vi "nRF52 DK Generate Packets.vi"() -> ()   [LabVIEW 2026, in "Nordic nRF52 DK DTM Test.lvlib"]
uses:
  Nordic nRF52 DK DTM Test.lvlib
  PacketType.ctl
  TxRx.ctl
panel:
  out "error out":errorcluster
  in  "stop":bool
  in  "Tx Packet Type":T1
  in  "BLE Channel Number (0-39)":u8
  in  "Com Port Resource":refnum<visa-resource-name>="COM3"
  in  "Baud Rate":u32=19200
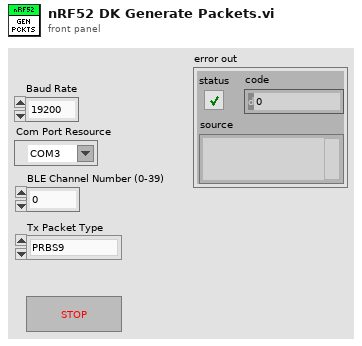
[diagram p1: front panel]
types:
  T1 = typedef "Nordic nRF52 DK DTM Test.lvlib/PacketType.ctl" = enum16{"PRBS9", "DF1", "DF2"}
  T2 = typedef "Nordic nRF52 DK DTM Test.lvlib/TxRx.ctl" = enum16{"Tx", "Rx"}
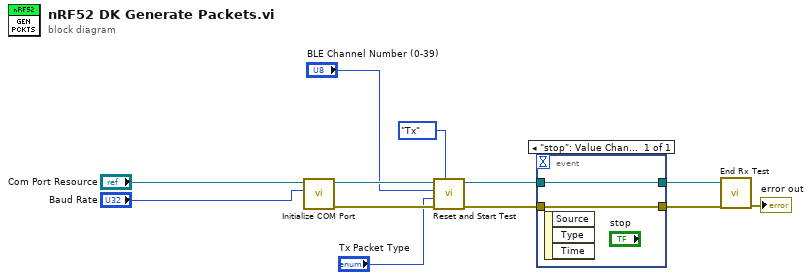
[diagram p0: block diagram]
diagram:
  n1 = call "Initialize COM Port.vi"("baud rate (9600)"="Baud Rate", "VISA Refnum in"="Com Port Resource") -> ("error out"=w8:errorcluster, "VISA Refnum out"=w9:refnum<visa-resource-name>)  [unwired: 8 in]
  n2 = call "Reset and Start Test.vi"("Tx/Rx"=TxRx."Tx", "error in (no error)"=w8, "Tx Packet Type"="Tx Packet Type", "BLE Channel Number (0-39)"="BLE Channel Number (0-39)", "VISA Refnum in"=w9) -> ("error out"=w5:errorcluster, "VISA Refnum out"=w4:refnum<visa-resource-name>)  [unwired: 4 in, 1 out]
  n3 = event shown="[0] \"stop\": Value Change" {
    selector: _ -> [_]
    dyn-events: _ -> [_]
    timeout: _ -> [_]
    tunnel: w5 -> [w13]
    tunnel: w4 -> [w14]
    tunnel: [w14] -> w3
    tunnel: [w13] -> w2
    event "stop": Value Change {
      n4 = event-data() -> ()  [unwired: 1 in, 3 out]
    }
  }
  n5 = call "End Rx Test.vi"("error in (no error)"=w2, "VISA Refnum in"=w3) -> ("error out"=→"error out":errorcluster)  [unwired: 7 in, 2 out]
